vi "globalTearDown.vi"(8 "error in":errorcluster, 11 "Multiple Instances in":refnum<class "Multiple Instances.lvclass">) -> (0 "error out":errorcluster, 3 "Multiple Instances out":refnum<class "Multiple Instances.lvclass">)   [LabVIEW 2020, in "Multiple Instances.lvclass"]
uses:
  Multiple Instances.lvclass
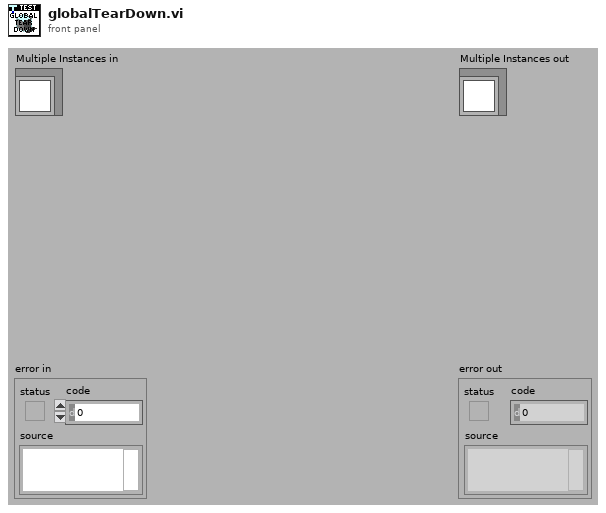
[diagram p1: front panel]
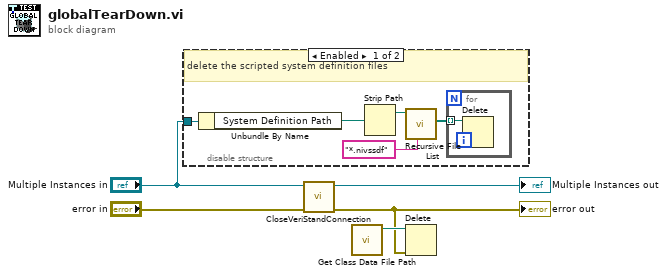
[diagram p0: block diagram]
diagram:
  n1 = disable-structure shown="Enabled" {
    disable-tunnel: "Multiple Instances in" -> [w10 _]
    frame Enabled {
      # "delete the scripted system definition files"
      n2 = Unbundle By Name(w10) -> ("System Definition Path"=w7:path)
      n3 = Strip Path(path=w7) -> (stripped path=w6:path)  [unwired: 1 out]
      n4 = call <vilib>:"Recursive File List.vi"("pattern"="*.nivssdf", "Folder Path"=w6) -> ("All Files in Dir"=w8:path[])  [unwired: 5 in, 4 out]
      n5 = for {
        tunnel: w8 -> [w11] mode=indexing
        n6 = Delete(path (use dialog)=w11) -> ()  [unwired: 4 in, 3 out]
      }
    }
    frame Disabled {
    }
  }
  n7 = call-dynamic "CloseVeriStandConnection.vi"("error in (no error)"="error in", "VeriStand Test Case in"="Multiple Instances in") -> ("error out"=w1:errorcluster, "VeriStand Test Case out"=→"Multiple Instances out":refnum<class "Multiple Instances.lvclass">)  [unwired: 8 in]
  "error out" <- w1
  n8 = call "Get Class Data File Path.vi"() -> ("Class Data File Path"=w5:path)  [unwired: 11 in]
  n9 = Delete(path (use dialog)=w5, error in=w1) -> ()  [unwired: 3 in, 3 out]
